vi "Start Acquisition.vi"(8 "error in (no error)":errorcluster, 10 "Continuous":bool, 11 "TDMS Data Source in":refnum<class "TDMS Data Source.lvclass">) -> (0 "error out":errorcluster, 3 "TDMS Data Source out":refnum<class "TDMS Data Source.lvclass">)   [LabVIEW 2020, in "TDMS Data Source.lvlib" / "TDMS Data Source.lvclass"]
uses:
  TDMS Data Source.lvclass
  C:/Program Files/National Instruments/LabVIEW 2026/vi.lib/ActorFramework/Actor/Actor.lvclass
  TDMS Data Source.lvclass/TDMS Data Source.ctl
  <vilib>/ActorFramework/Actor/Actor.lvclass/Actor.ctl
  <vilib>/ActorFramework/Message Enqueuer/Message Enqueuer.lvclass/Message Enqueuer.ctl
  TDMS Data Source Messages/Start Reading File Msg/Start Reading File Msg.lvclass/Start Reading File Msg.ctl
  <vilib>/ActorFramework/Message Enqueuer/Init from Existing Queue.vi
  <vilib>/ActorFramework/Message Enqueuer/Enqueue.vi
  TDMS Data Source Messages/Start Reading File Msg/Start Reading File Msg.lvclass
  C:/Program Files/National Instruments/LabVIEW 2026/vi.lib/ActorFramework/Message/Message.lvclass
  <vilib>/ActorFramework/Message Priority Queue/Priority Enqueue.vi
  <vilib>/ActorFramework/Message Enqueuer/Message Enqueuer.lvclass
  Data Source/Data Source/Data Source.lvclass
  <vilib>/ActorFramework/Actor/Actor.lvclass
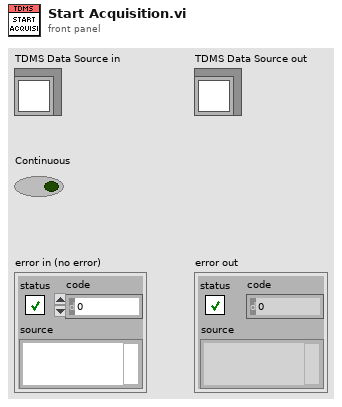
[diagram p1: front panel]
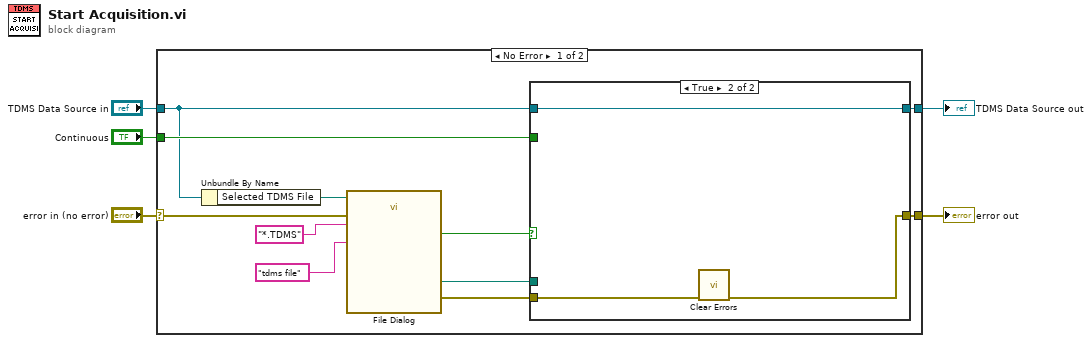
[diagram p0: block diagram]
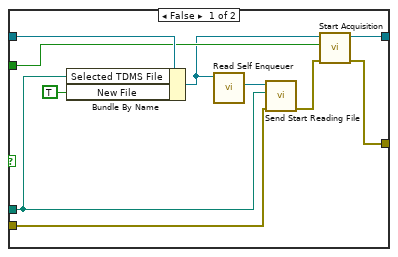
[diagram p2: hidden frame]
diagram:
  n1 = case shown="No Error" "error in (no error)" {
    selector: "error in (no error)" -> [w13 w31]
    tunnel: [w15 w31] -> w4
    tunnel: [w16 w30] -> w2
    tunnel: "TDMS Data Source in" -> [w10 w30]
    tunnel: "Continuous" -> [w14 _]
    frame No Error {
      n2 = Unbundle By Name(w10) -> ("Selected TDMS File"=w9:path)
      n3 = call "File Dialog"("start path"=w9, "button label"="tdms file", "error in"=w13, "pattern (all files)"="*.TDMS") -> ("selected path"=w6:path, "cancelled"=w11:bool, "error out"=w12:errorcluster)  [unwired: 8 in, 1 out]
      n4 = case shown="True" w11 {
        tunnel: w10 -> [w26 w29]
        tunnel: [w25 w29] -> w16
        tunnel: [w24 w27] -> w15
        tunnel: w14 -> [w23 _]
        tunnel: w12 -> [w19 w28]
        tunnel: w6 -> [w18 _]
        frame False {
          n5 = Bundle By Name(cluster=w26, "Selected TDMS File"=w18, "New File"=TRUE) -> (w22:refnum<class "TDMS Data Source.lvclass">)
          n6 = call <vilib>:"Read Self Enqueuer.vi"("Actor"=w22) -> ("Self Enqueuer"=w21:refnum<class "Message Enqueuer.lvclass">)  [unwired: 10 in]
          n7 = call "Send Start Reading File.vi"("error in (no error)"=w19, "TDMS File"=w18, "Message Enqueuer"=w21) -> ("error out"=w20:errorcluster)  [unwired: 7 in, 1 out]
          n8 = call-parent "Start Acquisition.vi"("error in (no error)"=w20, "Continuous"=w23, "Data Source in"=w22) -> ("error out"=w24:errorcluster, "Data Source out"=w25:refnum<class "TDMS Data Source.lvclass">)  [unwired: 7 in]
        }
        frame True {
          n9 = call <vilib>:"Clear Errors.vi"("error in (no error)"=w28) -> ("error out"=w27:errorcluster)  [unwired: 5 in, 1 out]
        }
      }
    }
    frame Error {
    }
  }
  "error out" <- w4
  "TDMS Data Source out" <- w2
